vi "Get Output Channel Values.vi"(11 "Output Process in":refnum<class "Output Process.lvclass">) -> (2 "Output Channel Values":dbl[](array[numeric]), 3 "Output Process out":refnum<class "Output Process.lvclass">)   [LabVIEW 2019, in "TelemetryAsync Engine.lvlib" / "Output Process.lvclass"]
uses:
  Output Process.lvclass
  Output Process.lvclass/Output Process.ctl
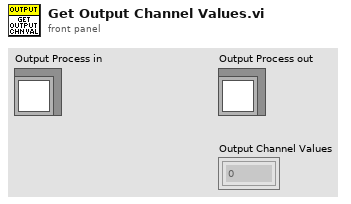
[diagram p1: front panel]
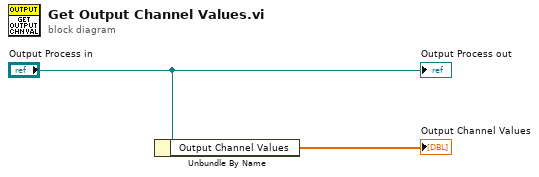
[diagram p0: block diagram]
diagram:
  n1 = Unbundle By Name("Output Process in") -> ("Output Channel Values"=→"Output Channel Values":dbl[])
  "Output Process out" <- "Output Process in"
